vi "Setup TS DAC.vi"(8 "error in":errorcluster, 11 "LNG Boiling Test Stand in":refnum<class "LNG Boiling Test Stand.lvclass">) -> (0 "error out":errorcluster, 3 "LNG Boiling Test Stand out":refnum<class "LNG Boiling Test Stand.lvclass">)   [LabVIEW 2019, in "Test Stands.lvlib" / "LNG Boiling Test Stand.lvclass"]
uses:
  LNG Boiling Test Stand.lvclass
  C:/Users/wg/Documents/LV_Projects/TestStand/App/Generic Test Stand/Generic Test Stand.lvclass
  DAC/LNG Boiling/Heater Box Temperatures/DAC Heater Box Temperatures.lvclass
  C:/Users/wg/Documents/LV_Projects/TestStand/App/DAC/DAC.lvclass
  DAC/DAC.lvclass
  DAC/LNG Boiling/Shunt dU/DAC Shunt dU.lvclass
  DAC/LNG Boiling/Heater dU/DAC Heater dU.lvclass
  DAC/LNG Boiling/Heater Ctrl/DAC Heater Ctrl.lvclass
  DAC/DAC.lvclass/DAC.ctl
  Generic Test Stand/Generic Test Stand.lvclass/Generic Test Stand.ctl
  Generic Test Stand/Generic Test Stand.lvclass
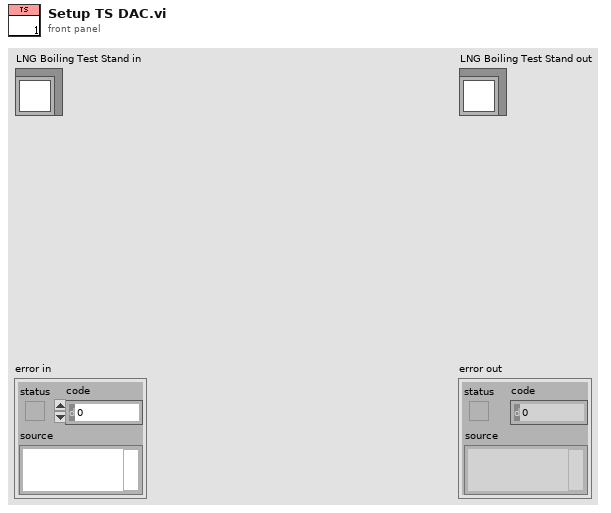
[diagram p1: front panel]
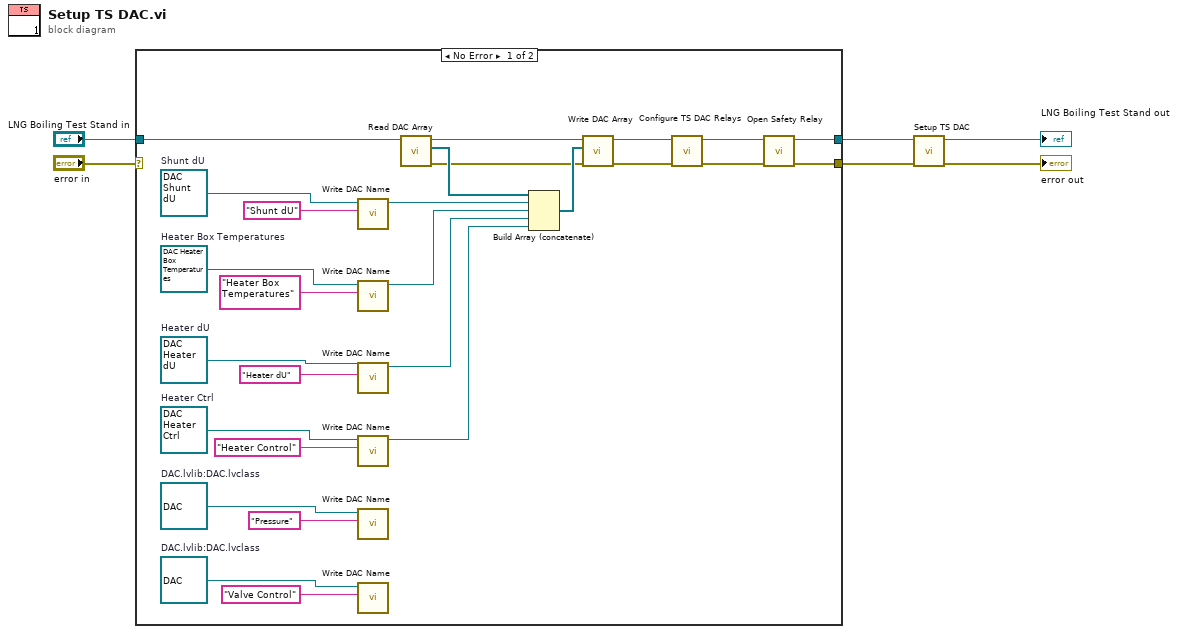
[diagram p0: block diagram]
diagram:
  n1 = case shown="No Error" "error in" {
    selector: "error in" -> [_ w34]
    tunnel: "LNG Boiling Test Stand in" -> [w28 w35]
    tunnel: [w12 w35] -> w2
    tunnel: [w9 w34] -> w1
    frame No Error {
      w7 = refnum<class "DAC Heater Ctrl.lvclass"> refnum  # Heater Ctrl
      w15 = refnum<class "DAC Heater dU.lvclass"> refnum  # Heater dU
      w17 = refnum<class "DAC Shunt dU.lvclass"> refnum  # Shunt dU
      w19 = refnum<class "DAC.lvclass"> refnum  # DAC.lvlib:DAC.lvclass
      w20 = refnum<class "DAC.lvclass"> refnum  # DAC.lvlib:DAC.lvclass
      w29 = refnum<class "DAC Heater Box Temperatures.lvclass"> refnum  # Heater Box Temperatures
      n2 = call "Write DAC Name.vi"("DAC Name"="Shunt dU", "DAC in"=w17) -> ("DAC out"=w23:refnum<class "DAC Shunt dU.lvclass">)  [unwired: 8 in, 1 out]
      n3 = call "Write DAC Name.vi"("DAC Name"="Heater Box Temperatures", "DAC in"=w29) -> ("DAC out"=w22:refnum<class "DAC Heater Box Temperatures.lvclass">)  [unwired: 8 in, 1 out]
      n4 = call "Write DAC Name.vi"("DAC Name"="Heater dU", "DAC in"=w15) -> ("DAC out"=w16:refnum<class "DAC Heater dU.lvclass">)  [unwired: 8 in, 1 out]
      n5 = call "Write DAC Name.vi"("DAC Name"="Heater Control", "DAC in"=w7) -> ("DAC out"=w8:refnum<class "DAC Heater Ctrl.lvclass">)  [unwired: 8 in, 1 out]
      n6 = call "Write DAC Name.vi"("DAC Name"="Pressure", "DAC in"=w20) -> ()  [unwired: 8 in, 2 out]
      n7 = call "Write DAC Name.vi"("DAC Name"="Valve Control", "DAC in"=w19) -> ()  [unwired: 8 in, 2 out]
      n8 = call "Read DAC Array.vi"("Generic Test Stand in"=w28) -> ("error out"=w24:errorcluster, "DAC Array"=w27:refnum<class "DAC.lvclass">[], "Generic Test Stand out"=w26:refnum<class "LNG Boiling Test Stand.lvclass">)  [unwired: 8 in]
      n9 = Build Array (concatenate)(w27, w23, w22, w16, w8) -> (w25:refnum<class "DAC.lvclass">[])
      n10 = call "Write DAC Array.vi"("error in (no error)"=w24, "DAC Array"=w25, "Generic Test Stand in"=w26) -> ("error out"=w11:errorcluster, "Generic Test Stand out"=w14:refnum<class "LNG Boiling Test Stand.lvclass">)  [unwired: 7 in]
      n11 = call "Configure TS DAC Relays.vi"("error in"=w11, "LNG Boiling Test Stand in"=w14) -> ("error out"=w10:errorcluster, "LNG Boiling Test Stand out"=w13:refnum<class "LNG Boiling Test Stand.lvclass">)  [unwired: 8 in]
      n12 = call "Open Safety Relay.vi"("error in (no error)"=w10, "LNG Boiling Test Stand in"=w13) -> ("error out"=w9:errorcluster, "LNG Boiling Test Stand out"=w12:refnum<class "LNG Boiling Test Stand.lvclass">)  [unwired: 8 in]
    }
    frame Error {
    }
  }
  n13 = call-parent "Setup TS DAC.vi"("error in (no error)"=w1, "Generic Test Stand in"=w2) -> ("error out"=→"error out":errorcluster, "Generic Test Stand out"=→"LNG Boiling Test Stand out":refnum<class "LNG Boiling Test Stand.lvclass">)  [unwired: 8 in]
